vi "IMAQ-MWT HT TEST (FPGA).vi"() -> ()   [LabVIEW 2015]
uses:
  <vilib>/Platform/TimedLoop/XDataNode/timing_clust.ctl
  <vilib>/Platform/TimedLoop/XDataNode/nitl_modes.ctl
  <vilib>/Platform/TimedLoop/XDataNode/wakeup.ctl
  <vilib>/rvi/Emulation/niFpgaSctlEmulationGetInTimedLoop.vi
  <vilib>/rvi/Emulation/niFpgaEmulationReportErrorSimple.vi
  <vilib>/rvi/Emulation/niFpgaGetClockAttributes.vi
  <vilib>/rvi/Emulation/niFpgaCriticalErrorInLSC.vi
  <vilib>/rvi/interface/RandomDataEmulation/niFpgaRandomDataHandleErrors.vi
  <vilib>/Platform/TimedLoop/XDataNode/XDataNode.xnode
  <vilib>/rvi/DataTransferAndStorage/Container/XNode/niFpgaContainer.xnode
  <vilib>/rvi/interface/RandomDataEmulation/nirviRandomDataFpgaReadWriteTemplate.vi
  <vilib>/Platform/TimedLoop/XDataNode/XDNodeRunTimeDep.lvlib
panel:
  out "Mean Angle":fxp<+/-,32,16> format="%.21g"
  in  "Scan End?":bool
  out "V1 (ID)":u16
  out "V2 (ID)":u16
  out "N Points":u16
  # "IMAQ - MWT"
  # "Camera Link Configuration"
  # "Camera Link Serial"
  # "Object Detection"
  # "Acquisition Settings"
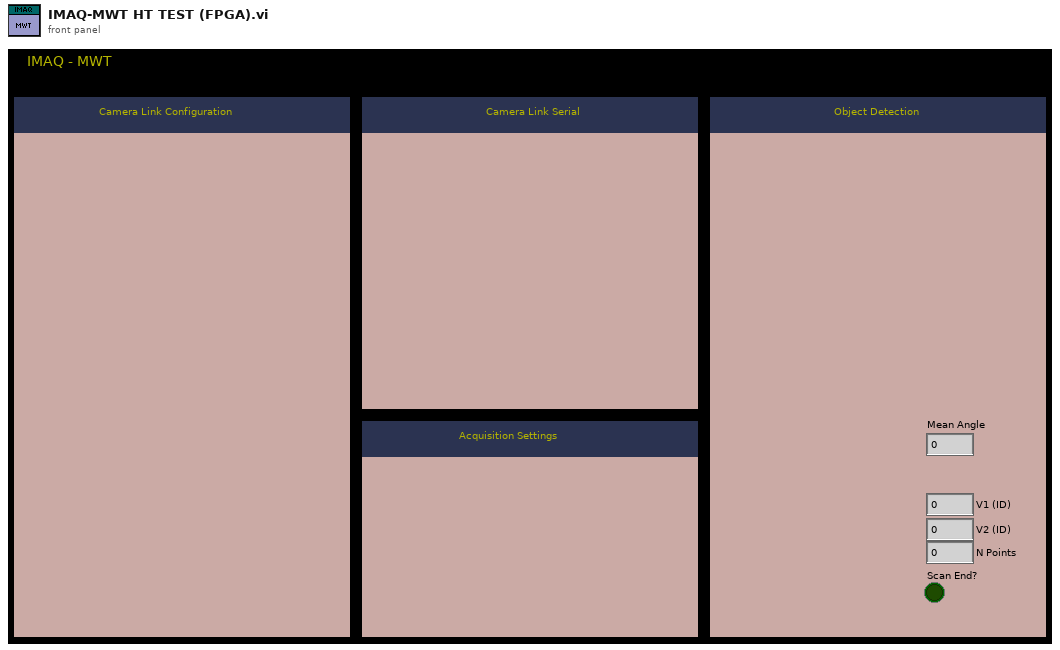
[diagram p1: front panel]
types:
  T1 = typedef "XDNodeRunTimeDep.lvlib/timing_clust.ctl" = cluster{"Expected End [f-1]":u64, "Actual End [f-1]":u64, "Finished Late? [f-1]":bool, "Expected End [i-1]":u64, "Actual End [i-1]":u64, "Finished Late? [i-1]":bool, "Expected Start [i]":u64, "Actual Start [i]":u64, "Expected Start [f]":u64, "Actual Start [f]":u64, "Source Name":string, "Structure Name":string, "Period":i64, "Deadline":i64, "Offset":i64, "Start":i64, "Priority":i32, "Timeout":i32, "Mode":T2, "Wakeup Reason":T3, "Error":errorcluster, "Source Type":string, "Secondary Source Type":string, "Global End Time":u64, "Global Start Time":u64, "Frame Duration":u64, "Iteration Duration":u64, "Assigned CPU":i32, "I/O Scan Engine Mode":u32}
  T2 = typedef "XDNodeRunTimeDep.lvlib/nitl_modes.ctl" = enum32{"No Change", "Process missed periods, maintain original phase", "Discard missed periods, maintain original phase", "Process missed periods, ignore original phase", "Discard missed periods, ignore original phase"}
  T3 = typedef "XDNodeRunTimeDep.lvlib/wakeup.ctl" = enum32{"Normal", "Aborted", "Asynchronous wakeup", "Timing source error", "Timed loop error", "Timeout"}
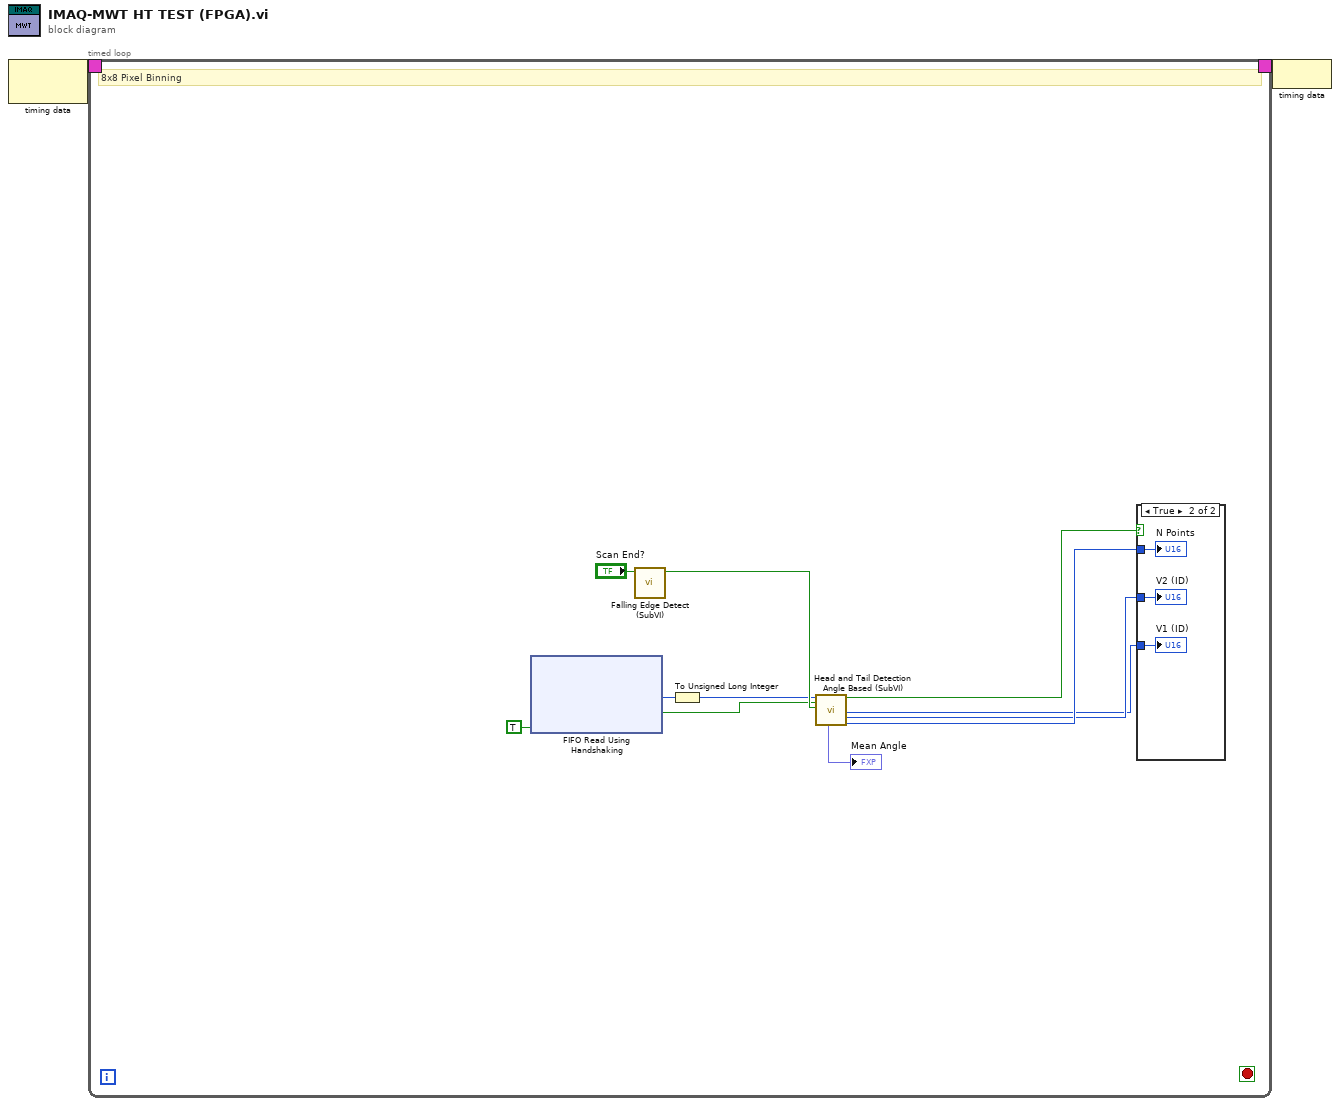
[diagram p0: block diagram]
diagram:
  n1 = node-c288() -> (w2:T1)  [unwired: 1 in]
  n2 = timed-loop {
    timing: w2 -> [_]
    timing-out: [_] -> w1
    stop <- _ stop-if-true
    # "8x8 Pixel Binning"
    n3 = xnode ("FIFO Read Using Handshaking")("Ready for Output"=TRUE) -> ("Element"=w8:u64, "Output Valid"=w4:bool)  [unwired: 1 in, 1 out]
    n4 = call "Falling Edge Detect (SubVI).vi"("Input"="Scan End?") -> ("Falling Edge?"=w6:bool)  [unwired: 10 in]
    n5 = To Unsigned Long Integer(number=w8) -> (unsigned 32bit integer=w5:u32)
    n6 = call "Head and Tail Detection Angle Based (SubVI).vi"("Boundary Point XY"=w5, "Bondary Valid?"=w4, "Scan End?"=w6) -> ("Mean Angle"=→"Mean Angle":fxp<+/-,32,16>, "Output Valid?"=w9:bool, "V1 (ID)"=w11:u16, "V2 (ID)"=w12:u16, "N Points"=w13:u16)  [unwired: 9 in, 3 out]
    n7 = case shown="True" w9 {
      tunnel: w13 -> [_ w16]
      tunnel: w12 -> [_ w15]
      tunnel: w11 -> [_ w14]
      frame False {
      }
      frame True {
        "N Points" <- w16
        "V2 (ID)" <- w15
        "V1 (ID)" <- w14
      }
    }
  }
  n8 = node-c288(w1) -> ()
